vi "nusic_note_index_by_noteoff_id.get.vi"(8 "error in (no error)":errorcluster, 11 "midi-ui in":refnum<class "midi-ui.lvclass">) -> (0 "error out":errorcluster, 2 "Music Note Index by NoteOffID":map{string, i32}(c390), 3 "midi-ui out":refnum<class "midi-ui.lvclass">)   [LabVIEW 2020, in "midi-ui.lvclass"]
uses:
  midi-ui.lvclass
  midi-ui.lvclass/midi-ui.ctl
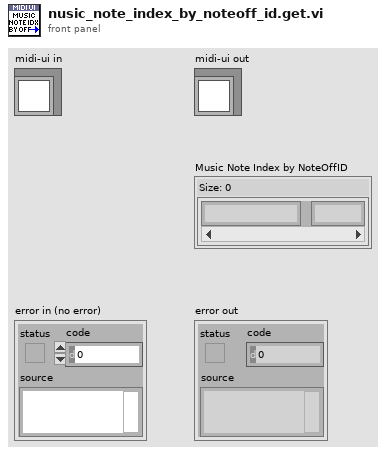
[diagram p1: front panel]
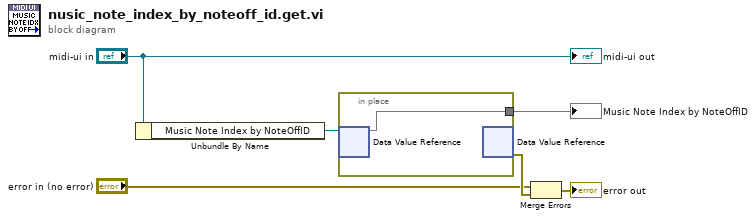
[diagram p0: block diagram]
diagram:
  n1 = Unbundle By Name("midi-ui in") -> ("Music Note Index by NoteOffID"=w6:refnum<data-value>)
  n2 = in-place {
    in-place-border: [w7] -> w1
    n3 = in-place-dvr #1(w6) -> (w7:map{string, i32})  [unwired: 1 out]
    n4 = in-place-dvr #1() -> (w4:errorcluster)  [unwired: 1 in, 1 out]
  }
  "Music Note Index by NoteOffID" <- w1
  n5 = Merge Errors("error in (no error)", w4) -> (→"error out":errorcluster)
  "midi-ui out" <- "midi-ui in"
